vi "DashboardCell2 Array Resize.vi"(5 "NumCols":i16, 6 "Cluster":T2={"Label Font Size"=24, "Data Font Size"=36, "String Font Size"=36}, 7 "NumRows":i16, 8 "error in":errorcluster, 9 "area height":i16, 10 "area width":i16, 11 "Array 2":refnum<vi>) -> (0 "error out":errorcluster)   [LabVIEW 2014, in "jkism-tool-support.lvlib"]
uses:
  jkism-tool-support.lvlib
panel:
  out "引气压力P4 2":T1={"Label"="Label", "Value"="0.00", "String"="0.00"} caption="Digital"
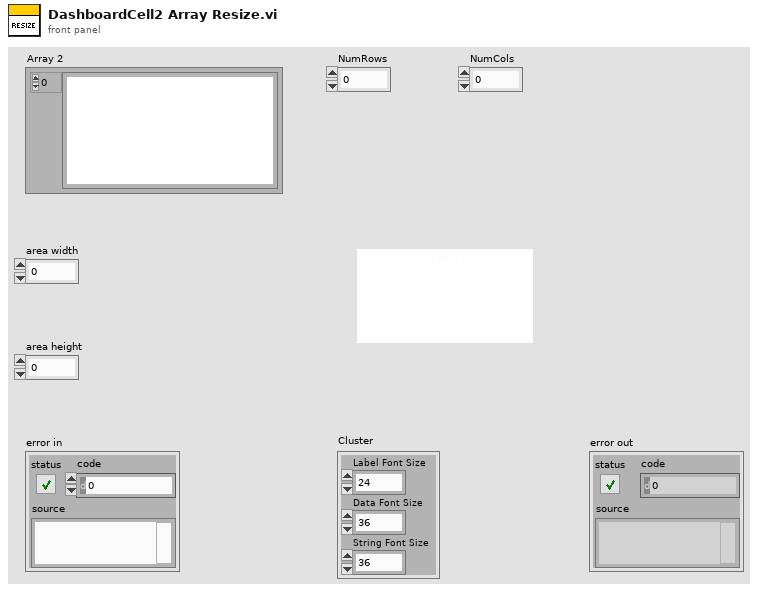
[diagram p1: front panel]
types:
  T1 = cluster{"Label":string, "Value":string, "String":string}
  T2 = cluster{"Label Font Size":i32, "Data Font Size":i32, "String Font Size":i32}
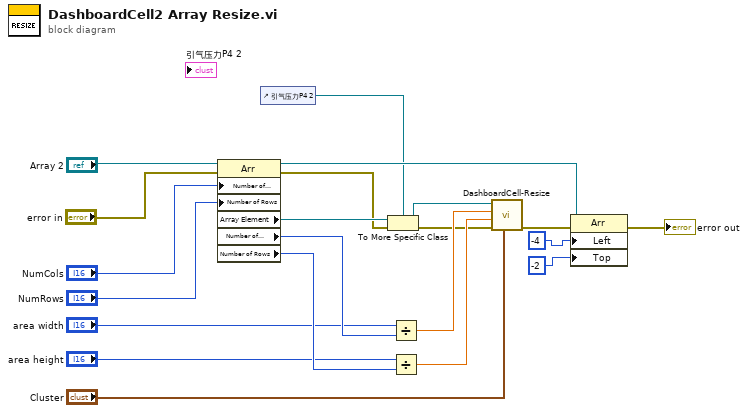
[diagram p0: block diagram]
diagram:
  n1 = property on="Property Node" class="Arr"(reference="Array 2", error in="error in", "Number of Columns"="NumCols", "Number of Rows"="NumRows") -> (reference out=w19:refnum<vi>, error out=w18:errorcluster, "Array Element"=w21:refnum<vi>, "Number of Columns"=w20:u32, "Number of Rows"=w17:u32)
  n2 = control-ref of="引气压力P4 2"() -> (w1:refnum<vi>)
  n3 = To More Specific Class(target class=w1, reference=w21, error in=w18) -> (specific class reference=w16:refnum<vi>, error out=w11:errorcluster)
  n4 = Divide(x="area width", y=w20) -> (x/y=w14:dbl)
  n5 = Divide(x="area height", y=w17) -> (x/y=w13:dbl)
  n6 = call "DashboardCell-Resize.vi"("Cluster"="Cluster", "error in (no error)"=w11, "Cluster Size:Height"=w13, "Cluster Size:Width"=w14, "引气压力P4 4"=w16) -> ("error out"=w15:errorcluster)  [unwired: 4 in, 2 out]
  n7 = property on="Property Node" class="Arr"(reference=w19, error in=w15, "Left"=-4 ("Position:Left"), "Top"=-2 ("Position:Left")) -> (error out=→"error out":errorcluster)  [unwired: 1 out]
